vi "setfiresettings.vi"(6 "Save Setting Permanently? (F)":bool, 8 "error in (no error)":errorcluster, 10 "firesetting {}":T1, 11 "hObject":i32) -> (0 "error out":errorcluster, 2 "pSettings":T1, 3 "hObject Out":i32)   [LabVIEW 2018]
doc: "this vi writes the FIRE setting to the device.\n\n<B>Save Setting Permanently? (F)</B>: If <B>TRUE</B>, the settings are written to the EEPROM and will retain it when the device is rebooted, otherwise, the settings will be reset upon rebooting.\n\n12/21/2010 1.0.0 jyg\n- initial release"
uses:
  ctl firesetting.ctl
  icsneo40.dll
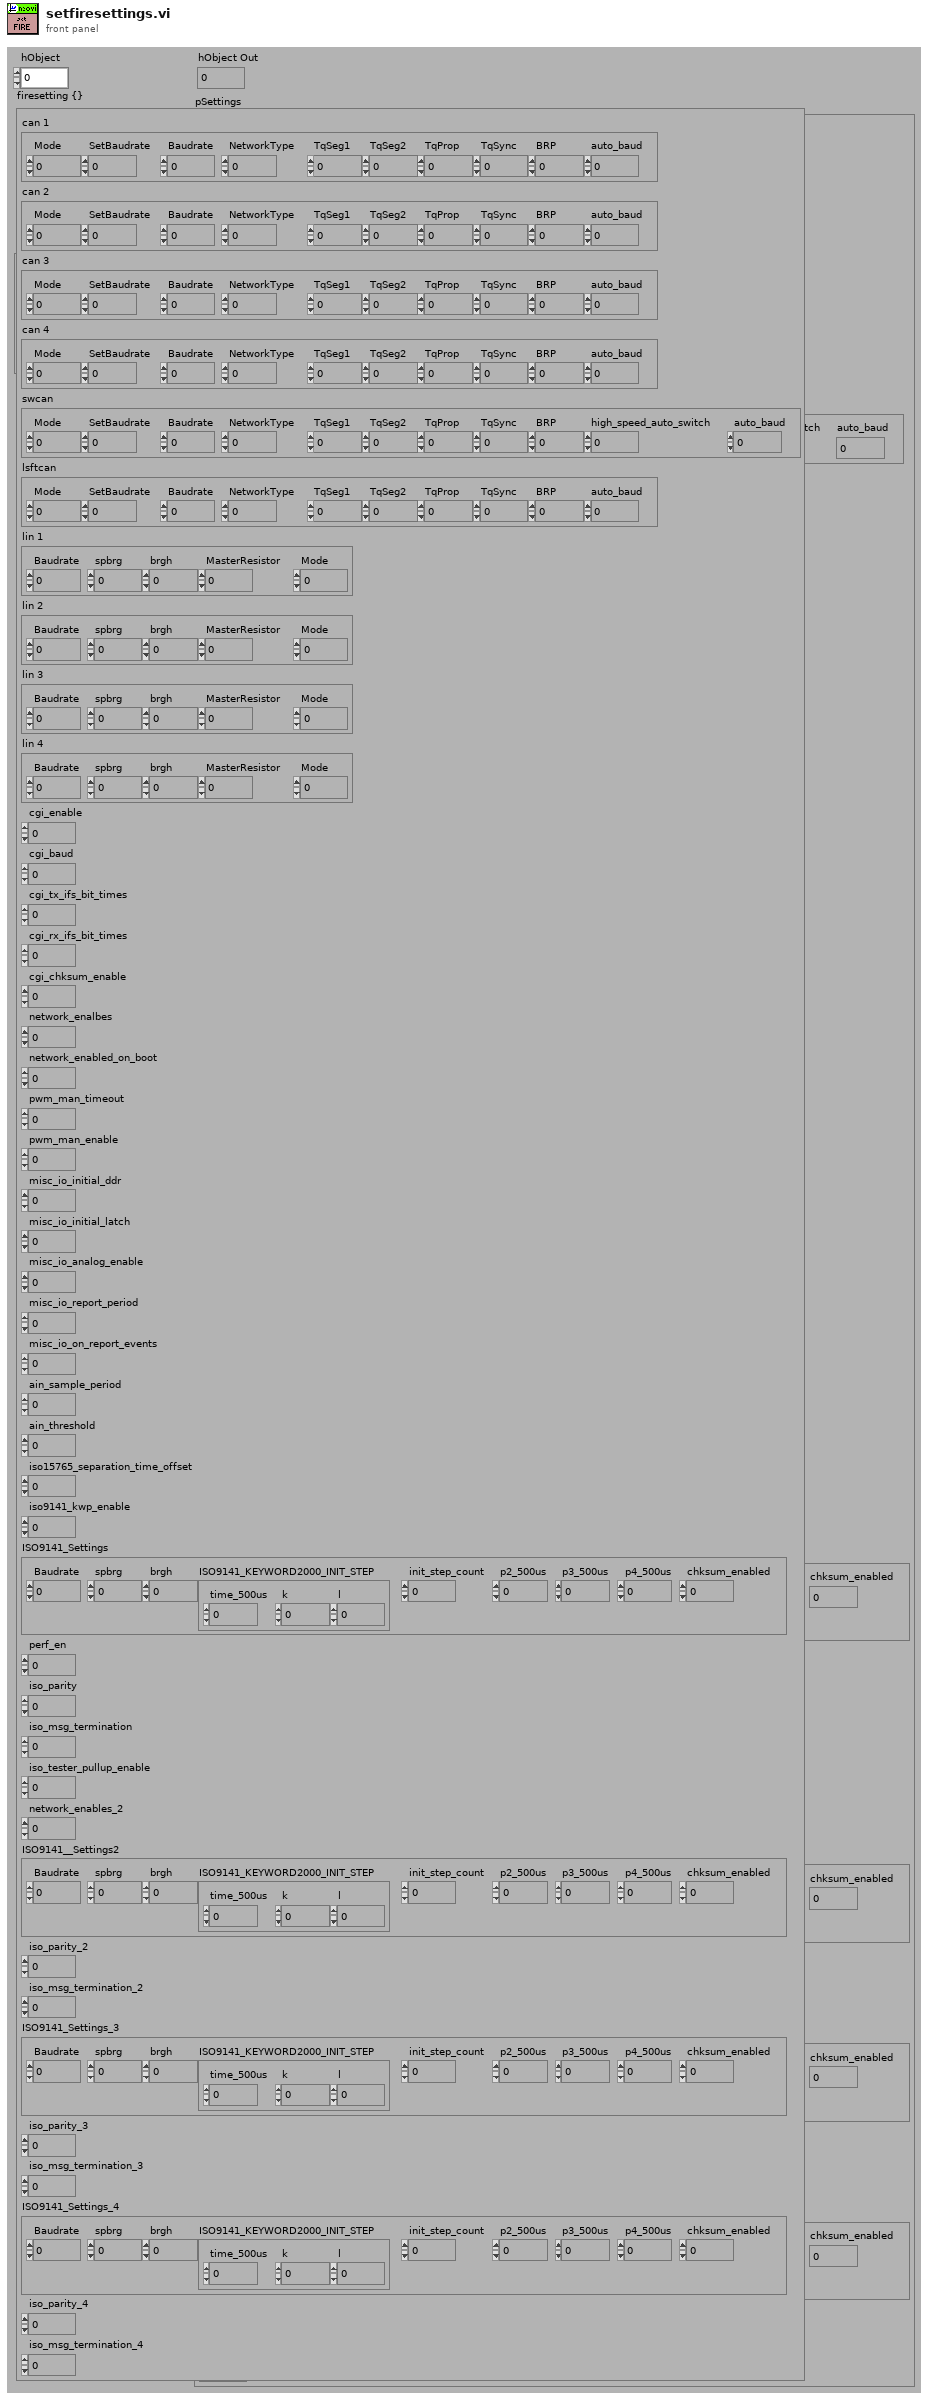
[diagram p1: front panel]
types:
  T1 = typedef "ctl FireSetting.ctl" = cluster{"can 1":cluster{"Mode":u8, "SetBaudrate":u8, "Baudrate":u8, "NetworkType":u8, "TqSeg1":u8, "TqSeg2":u8, "TqProp":u8, "TqSync":u8, "BRP":u16, "auto_baud":u16}, "can 2":cluster{"Mode":u8, "SetBaudrate":u8, "Baudrate":u8, "NetworkType":u8, "TqSeg1":u8, "TqSeg2":u8, "TqProp":u8, "TqSync":u8, "BRP":u16, "auto_baud":u16}, "can 3":cluster{"Mode":u8, "SetBaudrate":u8, "Baudrate":u8, "NetworkType":u8, "TqSeg1":u8, "TqSeg2":u8, "TqProp":u8, "TqSync":u8, "BRP":u16, "auto_baud":u16}, "can 4":cluster{"Mode":u8, "SetBaudrate":u8, "Baudrate":u8, "NetworkType":u8, "TqSeg1":u8, "TqSeg2":u8, "TqProp":u8, "TqSync":u8, "BRP":u16, "auto_baud":u16}, "swcan":cluster{"Mode":u8, "SetBaudrate":u8, "Baudrate":u8, "NetworkType":u8, "TqSeg1":u8, "TqSeg2":u8, "TqProp":u8, "TqSync":u8, "BRP":u16, "high_speed_auto_switch":u16, "auto_baud":u16}, "lsftcan":cluster{"Mode":u8, "SetBaudrate":u8, "Baudrate":u8, "NetworkType":u8, "TqSeg1":u8, "TqSeg2":u8, "TqProp":u8, "TqSync":u8, "BRP":u16, "auto_baud":u16}, "lin 1":cluster{"Baudrate":u32, "spbrg":u16, "brgh":u16, "MasterResistor":u8, "Mode":u8}, "lin 2":cluster{"Baudrate":u32, "spbrg":u16, "brgh":u16, "MasterResistor":u8, "Mode":u8}, "lin 3":cluster{"Baudrate":u32, "spbrg":u16, "brgh":u16, "MasterResistor":u8, "Mode":u8}, "lin 4":cluster{"Baudrate":u32, "spbrg":u16, "brgh":u16, "MasterResistor":u8, "Mode":u8}, "cgi_enable":u16, "cgi_baud":u16, "cgi_tx_ifs_bit_times":u16, "cgi_rx_ifs_bit_times":u16, "cgi_chksum_enable":u16, "network_enalbes":u16, "network_enabled_on_boot":u16, "pwm_man_timeout":u16, "pwm_man_enable":u16, "misc_io_initial_ddr":u16, "misc_io_initial_latch":u16, "misc_io_analog_enable":u16, "misc_io_report_period":u16, "misc_io_on_report_events":u16, "ain_sample_period":u16, "ain_threshold":u16, "iso15765_separation_time_offset":u16, "iso9141_kwp_enable":u16, "ISO9141_Settings":cluster{"Baudrate":u32, "spbrg":u16, "brgh":u16, "ISO9141_KEYWORD2000_INIT_STEP":cluster{"time_500us":u16, "k":u16, "l":u16}, "init_step_count":u8, "p2_500us":u16, "p3_500us":u16, "p4_500us":u16, "chksum_enabled":u16}, "perf_en":u16, "iso_parity":u16, "iso_msg_termination":u16, "iso_tester_pullup_enable":u16, "network_enables_2":u16, "ISO9141__Settings2":cluster{"Baudrate":u32, "spbrg":u16, "brgh":u16, "ISO9141_KEYWORD2000_INIT_STEP":cluster{"time_500us":u16, "k":u16, "l":u16}, "init_step_count":u8, "p2_500us":u16, "p3_500us":u16, "p4_500us":u16, "chksum_enabled":u16}, "iso_parity_2":u16, "iso_msg_termination_2":u16, "ISO9141_Settings_3":cluster{"Baudrate":u32, "spbrg":u16, "brgh":u16, "ISO9141_KEYWORD2000_INIT_STEP":cluster{"time_500us":u16, "k":u16, "l":u16}, "init_step_count":u8, "p2_500us":u16, "p3_500us":u16, "p4_500us":u16, "chksum_enabled":u16}, "iso_parity_3":u16, "iso_msg_termination_3":u16, "ISO9141_Settings_4":cluster{"Baudrate":u32, "spbrg":u16, "brgh":u16, "ISO9141_KEYWORD2000_INIT_STEP":cluster{"time_500us":u16, "k":u16, "l":u16}, "init_step_count":u8, "p2_500us":u16, "p3_500us":u16, "p4_500us":u16, "chksum_enabled":u16}, "iso_parity_4":u16, "iso_msg_termination_4":u16}
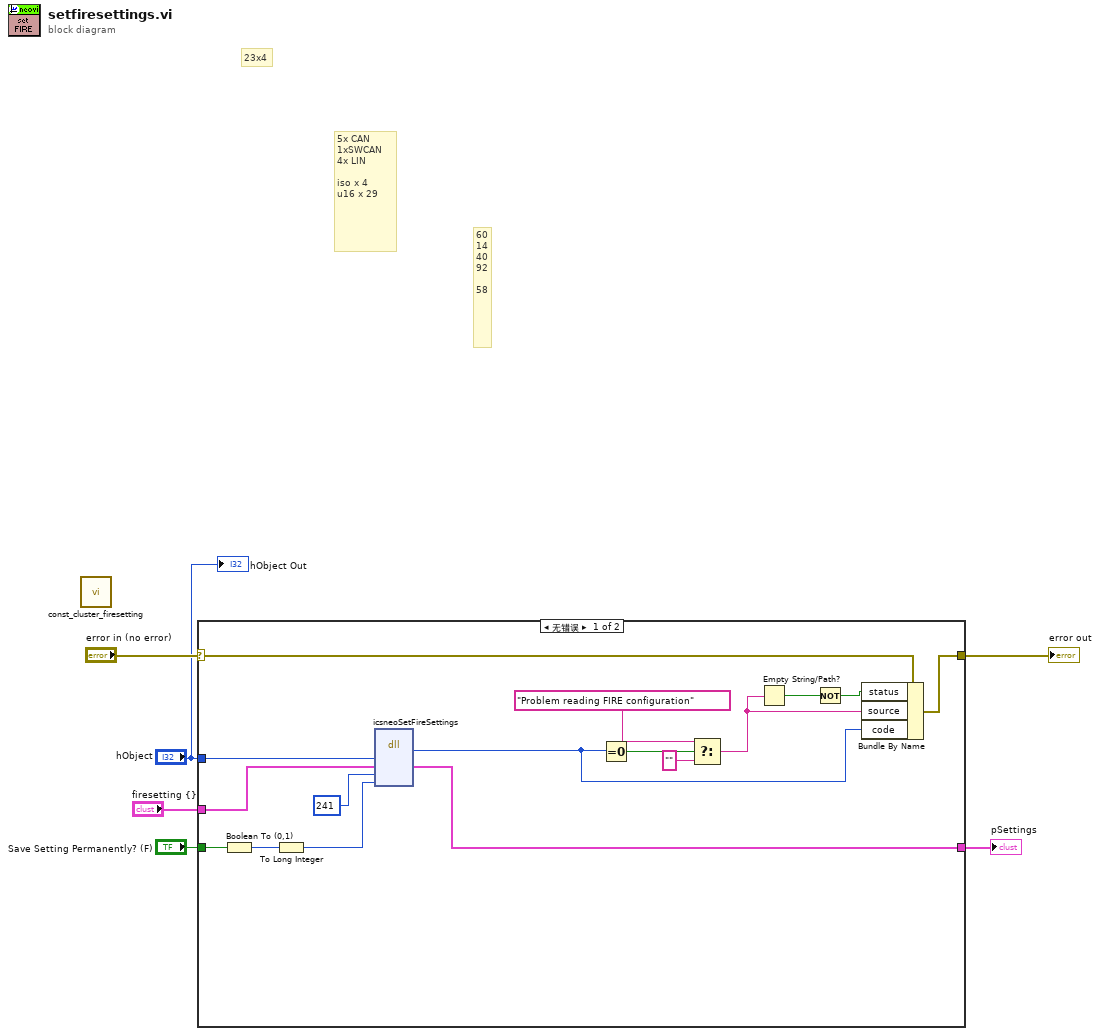
[diagram p0: block diagram]
diagram:
  # "23x4"
  # "60\n14\n40\n92\n\n58"
  # "5x CAN\n1xSWCAN\n4x LIN\n\niso x 4\nu16 x 29"
  n1 = call "const_cluster_firesetting.vi"() -> ()  [unwired: 1 out]
  n2 = case shown="无错误" "error in (no error)" {
    selector: "error in (no error)" -> [w18 w23]
    tunnel: [w19 w23] -> w6
    tunnel: "hObject" -> [w14 _]
    tunnel: "firesetting {}" -> [w13 _]
    tunnel: [w11 _] -> w3
    tunnel: "Save Setting Permanently? (F)" -> [w9 _]
    frame No Error {
      n3 = Boolean To (0,1)(Boolean=w9) -> (0, 1=w8:i16)
      n4 = To Long Integer(number=w8) -> (32bit integer=w7:i32)
      n5 = dll-call lib="icsneo40.dll" fn="icsneoSetFireSettings"("hObject"=w14, "pSettings"=w13, "iNumBytes"=241, "bSaveToEEPROM"=w7) -> ("return type"=w17:i32, "pSettings"=w11:T1)  [unwired: 6 in, 2 out]
      n6 = Equal To 0?(x=w17) -> (x = 0?=w16:bool)
      n7 = Select(t="Problem reading FIRE configuration", s=w16, f="") -> (s? t:f=w15:string)
      n8 = Empty String/Path?(string/path=w15) -> (empty?=w21:bool)
      n9 = Not(x=w21) -> (.not. x?=w20:bool)
      n10 = Bundle By Name(cluster=w18, "status"=w20, "source"=w15, "code"=w17) -> (w19:errorcluster)
    }
    frame Error {
    }
  }
  "error out" <- w6
  "pSettings" <- w3
  "hObject Out" <- "hObject"
